vi "PID.vi"(6 "State":dbl, 7 "Reference":dbl, 8 "PID vals in":cluster{"e_prev":dbl, "e_int":dbl}, 9 "Step_size":dbl, 10 "PID gains":T1, 11 "output range":cluster{"output high":dbl, "output low":dbl}) -> (2 "PID vals out":cluster{"e_prev":dbl, "e_int":dbl}, 3 "input":dbl)   [LabVIEW 2025, in "Dynamic-System.lvclass"]
uses:
  Dynamic-System.lvclass
  Dynamic-System.lvclass/Dynamic-System.ctl
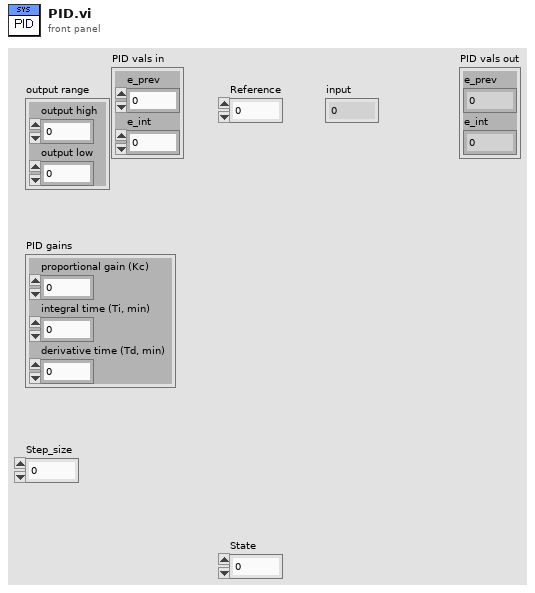
[diagram p1: front panel]
types:
  T1 = cluster{"proportional gain (Kc)":dbl, "integral time (Ti, min)":dbl, "derivative time (Td, min)":dbl}
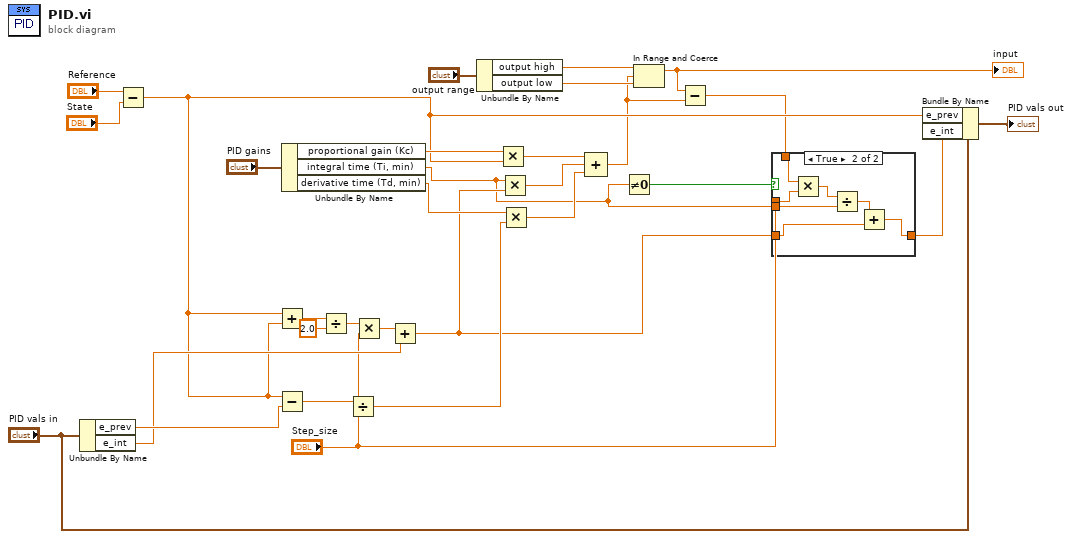
[diagram p0: block diagram]
diagram:
  n1 = Unbundle By Name("PID vals in") -> ("e_prev"=w19:dbl, "e_int"=w14:dbl)
  n2 = Subtract(x="Reference", y="State") -> (x-y=w9:dbl)
  n3 = Add(x=w9, y=w9) -> (x+y=w16:dbl)
  n4 = Subtract(x=w9, y=w19) -> (x-y=w18:dbl)
  n5 = Unbundle By Name("PID gains") -> ("proportional gain (Kc)"=w26:dbl, "integral time (Ti, min)"=w1:dbl, "derivative time (Td, min)"=w25:dbl)
  n6 = Divide(x=w16, y=2.0) -> (x/y=w13:dbl)
  n7 = Divide(x=w18, y="Step_size") -> (x/y=w17:dbl)
  n8 = Multiply(x=w13, y="Step_size") -> (x*y=w12:dbl)
  n9 = Add(x=w12, y=w14) -> (x+y=w7:dbl)
  n10 = Unbundle By Name("output range") -> ("output high"=w29:dbl, "output low"=w28:dbl)
  n11 = Multiply(x=w26, y=w9) -> (x*y=w24:dbl)
  n12 = Multiply(x=w1, y=w7) -> (x*y=w23:dbl)
  n13 = Multiply(x=w25, y=w17) -> (x*y=w22:dbl)
  n14 = Compound Arithmetic op=ADD(w24, w23, w22) -> (w4:dbl)
  n15 = Not Equal To 0?(x=w1) -> (x != 0?=w8:bool)
  n16 = In Range and Coerce(upper limit=w29, x=w4, lower limit=w28) -> (coerced(x)=w5:dbl)  [unwired: 1 out]
  "input" <- w5
  n17 = Subtract(x=w5, y=w4) -> (x-y=w3:dbl)
  n18 = case shown="True" w8 {
    tunnel: w7 -> [w31 w33]
    tunnel: [w31 w32] -> w6
    tunnel: w3 -> [_ w38]
    tunnel: "Step_size" -> [_ w37]
    tunnel: w1 -> [_ w35]
    frame False {
    }
    frame True {
      n19 = Multiply(x=w38, y=w37) -> (x*y=w36:dbl)
      n20 = Divide(x=w36, y=w35) -> (x/y=w34:dbl)
      n21 = Add(x=w34, y=w33) -> (x+y=w32:dbl)
    }
  }
  n22 = Bundle By Name(cluster="PID vals in", "e_prev"=w9, "e_int"=w6) -> (→"PID vals out":cluster{"e_prev":dbl, "e_int":dbl})
